vi "Run Test Cases in Suite.vi"(8 "error in (no error)":errorcluster, 10 "Test Suite":refnum<class "LUnit Test Suite.lvclass">, 11 "Test Runner In":refnum<class "Test Runner.lvclass">) -> (0 "error out":errorcluster, 3 "Test Runner Out":refnum<class "Test Runner.lvclass">)   [LabVIEW 2020, in "Test Runner.lvclass"]
uses:
  Test Runner.lvclass
  Test Suite/LUnit Test Suite.lvclass
  Test Runner.lvclass/Test Runner.ctl
  Test Suite/LUnit Test Suite.lvclass/LUnit Test Suite.ctl
  Application Framework/Process Classes/Process/Process.lvclass/Process.ctl
  Slave Test Runner/Slave Test Runner.lvclass/Slave Test Runner.ctl
  Test Case/LUnit Test Case.lvclass/LUnit Test Case.ctl
  Result Collector/Result Collector.lvclass/Result Collector.ctl
  Application Framework/Process Classes/Process/Protected/Messaging/Enqueue Message.vi
  Result Types/Suite Results/Public/Get Execution time.vi
  Result Collector/Public/API/Collect Suite Result.vi
  Build Schedule.vi
  Slave Test Runner/Public/API/Run Test Case.vi
  Result Types/Suite Results/Public/Aggregate Test Case Results.vi
  Result Types/Case Result/Public/Read Status.vi
  Result Types/Suite Results/Private/Merge Status.vi
  Result Types/Case Result/Private/Merge Status.vi
  Result Types/Method Result/Public/Read Status.vi
  Slave Test Runner/Slave Test Runner.lvclass
  C:/Git/astemes-lunit/source/Application Framework/Process Classes/Process/Process.lvclass
  Test Case/LUnit Test Case.lvclass
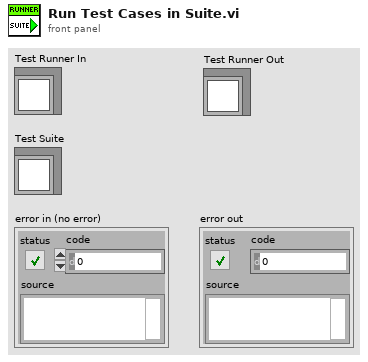
[diagram p1: front panel]
types:
  T1 = typedef "Test Case Result.lvlib/Test Case Result type.ctl" = map{string, T2}
  T2 = typedef "Method Result.lvlib/Method Result type.ctl" = cluster{"Test Case":string, "Test Method Name":string, "Status":T3, "Assertion Results":T4[], "Execution time":dbl, "Result String":string}
  T3 = typedef "Assertion Result.lvlib/Status.ctl" = enum16{"Pass", "Fail", "Error", "Skipped", "Setup Error", "Broken", "Teardown Error"}
  T4 = typedef "Assertion Result.lvlib/Assertion Result type.ctl" = cluster{"Status":T3, "Message":string, "Description":string, "Assertion Type":T5}
  T5 = typedef "Assertion Result.lvlib/Assertion Type.ctl" = enum16{"None", "Pass", "Fail", "Skip", "Pass if Equal", "Fail if Equal", "Pass if Error", "Fail if Error", "Pass if", "Fail if"}
  T6 = typedef "Test Suite Result.lvlib/Test Suite Result type.ctl" = cluster{"Test Suite ID":string, "Name":string, "Hostname":string, "Status":T3, "Execution time":dbl, "Start Time":timestamp, "Case Results":T1[]}
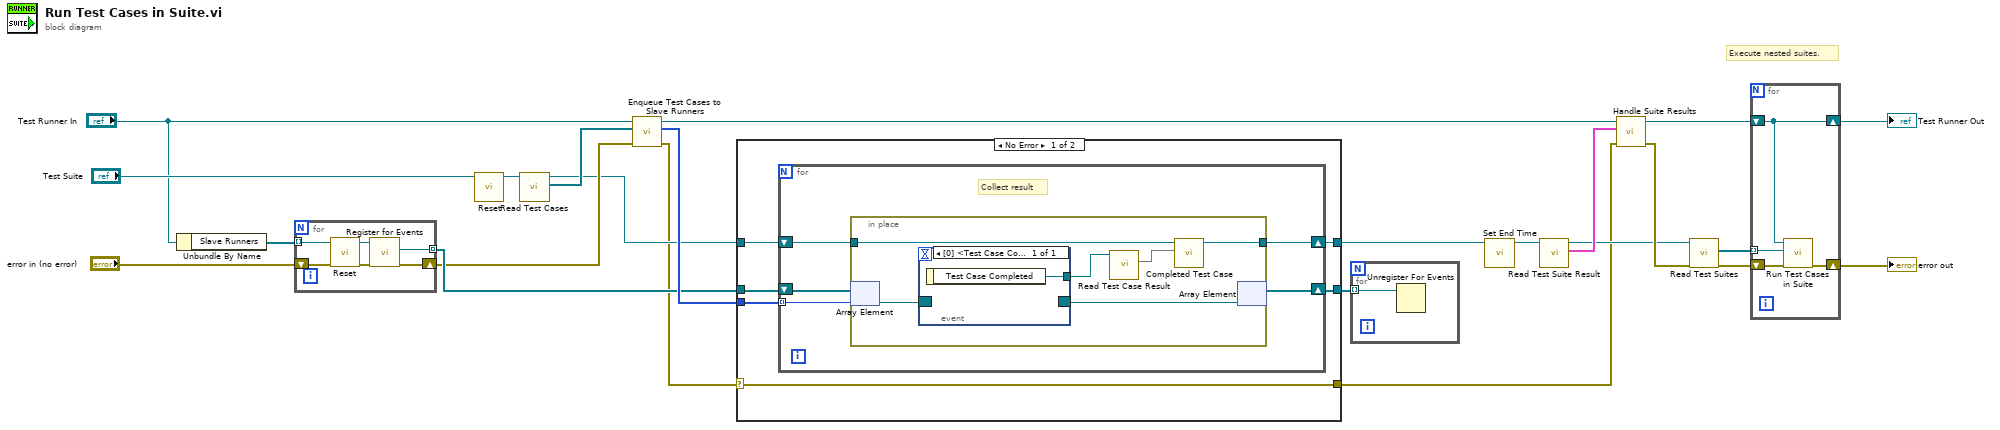
[diagram p0: block diagram]
diagram:
  # "Execute nested suites."
  n1 = Unbundle By Name("Test Runner In") -> ("Slave Runners"=w13:refnum<class "Slave Test Runner.lvclass">[])
  n2 = for {
    tunnel: w13 -> [w28] mode=indexing
    tunnel: [w30] -> w11 mode=indexing
    shift-right: [w29] -> w9
    shift-left: "error in (no error)" -> [w25]
    n3 = call "Reset.vi"("error in (no error)"=w25, "Slave Test Runner In"=w28) -> ("error out"=w26:errorcluster, "Slave Test Runner Out"=w27:refnum<class "Slave Test Runner.lvclass">)  [unwired: 8 in]
    n4 = call "Register for Events.vi"("error in (no error)"=w26, "Slave Test Runner In"=w27) -> ("error out"=w29:errorcluster, "Event Registration Refnum"=w30:refnum<event-registration>)  [unwired: 7 in, 1 out]
  }
  n5 = call "Reset.vi"("Test Suite In"="Test Suite") -> ("Test Suite Out"=w20:refnum<class "LUnit Test Suite.lvclass">)  [unwired: 10 in]
  n6 = call "Read Test Cases.vi"("Test Suite In"=w20) -> ("Test Cases"=w15:refnum<class "LUnit Test Case.lvclass">[], "Test Suite Out"=w8:refnum<class "LUnit Test Suite.lvclass">)  [unwired: 9 in]
  n7 = call "Enqueue Test Cases to Slave Runners.vi"("error in (no error)"=w9, "Test Cases"=w15, "Test Runner in"="Test Runner In") -> ("error out"=w4:errorcluster, "Schedule"=w12:i32[], "Test Runner out"=w10:refnum<class "Test Runner.lvclass">)  [unwired: 6 in]
  n8 = case shown="No Error" w4 {
    selector: w4 -> [w31 w49]
    tunnel: [w36 w50] -> w14
    tunnel: w12 -> [w35 _]
    tunnel: w11 -> [w34 w51]
    tunnel: w8 -> [w33 w50]
    tunnel: [w32 w51] -> w7
    tunnel: [w31 w49] -> w3
    frame No Error {
      n9 = for {
        shift-right: [w41] -> w36
        shift-left: w33 -> [w40]
        tunnel: w35 -> [w39] mode=indexing
        shift-right: [w37] -> w32
        shift-left: w34 -> [w38]
        # "Collect result"
        n10 = in-place {
          in-place-border: [w47] -> w41
          in-place-border: w40 -> [w46]
          n11 = in-place-array #1(w38, w39) -> (w43:refnum<event-registration>)
          n12 = event shown="[0] <Test Case Completed>: User Event" {
            selector: w43 -> [_]
            dyn-events: [_] -> w42
            timeout: _ -> [_]
            tunnel: [w48] -> w45
            event User Event {
              n13 = event-data() -> ("Test Case Completed"=w48:refnum<class "LUnit Test Case.lvclass">)  [unwired: 1 in]
            }
          }
          n14 = call "Read Test Case Result.vi"("LUnit Test Case In"=w45) -> ("Test Case Result"=w44:T1)  [unwired: 9 in, 1 out]
          n15 = call "Completed Test Case.vi"("Test Case Result"=w44, "Test Suite In"=w46) -> ("Test Suite Out"=w47:refnum<class "LUnit Test Suite.lvclass">)  [unwired: 9 in]
          n16 = in-place-array #1(w42) -> (w37:refnum<event-registration>[])  [unwired: 1 out]
        }
      }
    }
    frame Error {
    }
  }
  n17 = for {
    tunnel: w7 -> [w52] mode=indexing
    n18 = Unregister For Events(event registration refnum=w52) -> ()  [unwired: 1 in, 1 out]
  }
  n19 = call "Set End Time.vi"("Test Suite In"=w14) -> ("Test Suite Out"=w19:refnum<class "LUnit Test Suite.lvclass">)  [unwired: 10 in]
  n20 = call "Read Test Suite Result.vi"("Test Suite In"=w19) -> ("Test Suite Result"=w21:T6, "Test Suite Out"=w17:refnum<class "LUnit Test Suite.lvclass">)  [unwired: 9 in]
  n21 = call "Handle Suite Results.vi"("error in (no error)"=w3, "Test Suite Result"=w21, "Test Runner In"=w10) -> ("error out"=w18:errorcluster, "Test Runner Out"=w16:refnum<class "Test Runner.lvclass">)  [unwired: 7 in]
  n22 = call "Read Test Suites.vi"("error in (no error)"=w18, "Test Suite In"=w17) -> ("error out"=w2:errorcluster, "Test Suites"=w1:refnum<class "LUnit Test Suite.lvclass">[])  [unwired: 7 in, 1 out]
  n23 = for {
    shift-right: [w55] -> w23
    shift-left: w2 -> [w56]
    shift-right: [w53] -> w22
    shift-left: w16 -> [w53]
    tunnel: w1 -> [w54] mode=indexing
    n24 = call "Run Test Cases in Suite.vi"("error in (no error)"=w56, "Test Suite"=w54, "Test Runner In"=w53) -> ("error out"=w55:errorcluster)  [unwired: 7 in, 1 out]
  }
  "error out" <- w23
  "Test Runner Out" <- w22
